vi "Actor Core.vi"(8 "error in":errorcluster, 11 "ModelSynchronouslyRequestsDoubleFloat In":refnum<class "ModelSynchronouslyRequestsDoubleFloat.lvclass">) -> (0 "error out":errorcluster, 3 "Actor out":refnum<class "Actor.lvclass">)   [LabVIEW 2020, in "ModelSynchronouslyRequestsDoubleFloat.lvclass"]
doc: "(<B>Filename</B>: Actor Framework.lvlib:Actor.lvclass:Actor Core.vi)\n\nReceives messages to the actor, reacts to them, and initiates any error handling that may shut the actor down.\n\nDescendant classes may override this VI to append parallel tasks for the actor to complete while it handles messages. Overrides use the Call Parent Method node."
uses:
  ModelSynchronouslyRequestsDoubleFloat.lvclass
  ModelSynchronouslyRequestsDoubleFloat.lvclass/ModelSynchronouslyRequestsDoubleFloat.ctl
  e2aabd18-2fb0-4fe7-9022-e482d04c71d6.vi
  Source/IModel/IModel/IModel.lvclass
  <vilib>/ActorFramework/Actor/Actor.lvclass
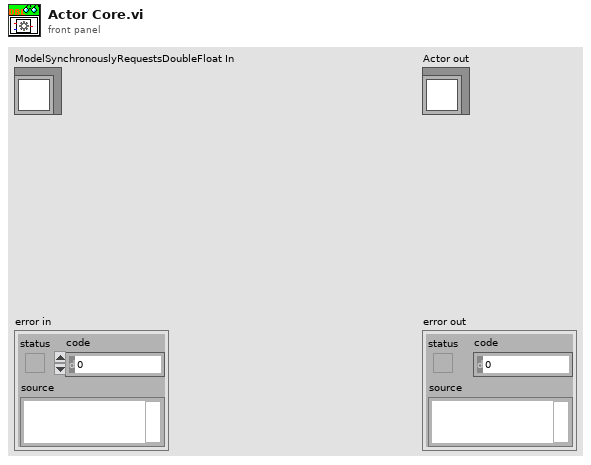
[diagram p1: front panel]
types:
  T1 = cluster{"Data":dbl, "timed out?":bool, "error out":errorcluster}
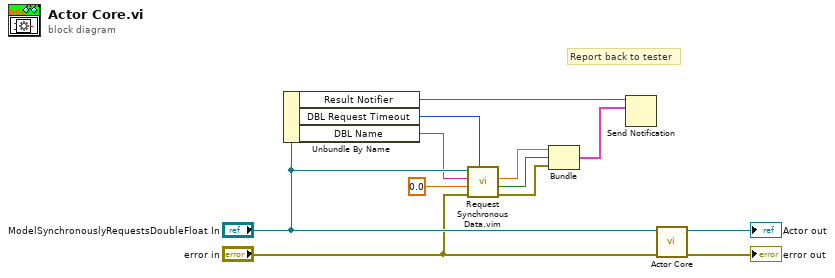
[diagram p0: block diagram]
diagram:
  # "Report back to tester"
  n1 = Unbundle By Name("ModelSynchronouslyRequestsDoubleFloat In") -> ("Result Notifier"=w10:refnum<notifier>, "DBL Request Timeout"=w5:i32, "DBL Name"=w8:string)
  n2 = call "Request Synchronous Data.vim"("Timeout In ms (-1)"=w5, "error in (no error)"="error in", "Type"=0.0, "Datum Name"=w8, "IObserver In"="ModelSynchronouslyRequestsDoubleFloat In") -> ("error out"=w2:errorcluster, "timed out?"=w3:bool, "Data"=w4:dbl)  [unwired: 3 in, 1 out]
  n3 = Bundle("Data"=w4, "timed out?"=w3, "error out"=w2) -> (w1:T1)  [unwired: 1 in]
  n4 = Send Notification(notification=w1, notifier=w10) -> ()  [unwired: 1 in, 2 out]
  n5 = call-parent "Actor Core.vi"("error in"="error in", "Actor in"="ModelSynchronouslyRequestsDoubleFloat In") -> ("error out"=→"error out":errorcluster, "Actor out"=→"Actor out":refnum<class "Actor.lvclass">)  [unwired: 8 in]
